vi "Create Instrument Addon From Configuration File.vi"(8 "error in (no error)":errorcluster, 10 "configuration file path":path, 11 "target in":refnum<k24>) -> (0 "error out":errorcluster, 2 "instrument addon refnum":T1=18446744073709551615 format="%.0x", 3 "target out":refnum<k24>)   [LabVIEW 2020, in "Instrument Addon Scripting API.lvlib"]
doc: "Creates an Instrument Addon and configures it according to the configuration file."
uses:
  Instrument Addon Scripting API.lvlib
  NationalInstruments.VeriStand.SystemDefinitionAPI
  <vilib>/NI VeriStand/Custom Device API/Custom Device Item Ref.ctl
  <vilib>/NI/NI VeriStand Custom Device Import and Export Tool/ImportExport.lvlib
  Addon/Addon Shared/Instrument Addon Shared.lvlib
  <vilib>/NI VeriStand/Custom Device API/Custom Device API.lvlib
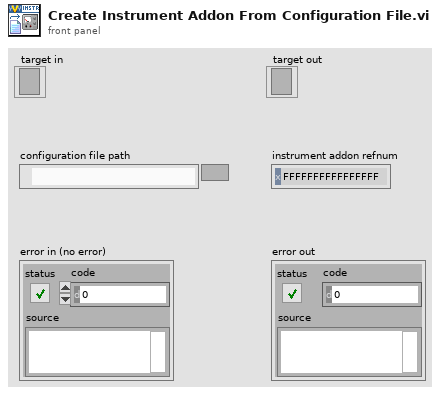
[diagram p1: front panel]
types:
  T1 = typedef "Custom Device API.lvlib/Custom Device Item Ref.ctl" = u64
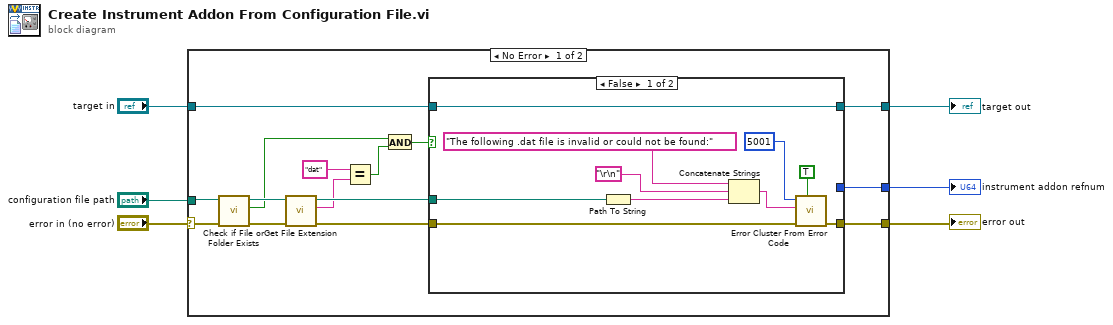
[diagram p0: block diagram]
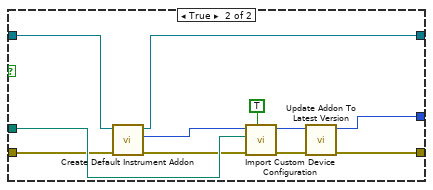
[diagram p2: hidden frame]
diagram:
  n1 = case shown="No Error" "error in (no error)" {
    selector: "error in (no error)" -> [w15 w44]
    tunnel: "target in" -> [w21 w43]
    tunnel: [w20 w43] -> w5
    tunnel: "configuration file path" -> [w13 _]
    tunnel: [w19 w44] -> w3
    tunnel: [w18 _] -> w1
    frame No Error {
      n2 = call <vilib>:"Check if File or Folder Exists.vi"("error in (no error)"=w15, "path"=w13) -> ("error out"=w14:errorcluster, "file or folder exists?"=w11:bool, "dup path"=w12:path)  [unwired: 7 in]
      n3 = call <vilib>:"Get File Extension.vi"("error in (no error)"=w14, "file"=w12) -> ("error out"=w17:errorcluster, "lowercase file extension"=w9:string, "dup file"=w16:path)  [unwired: 5 in, 2 out]
      n4 = Equal?(x="dat", y=w9) -> (x = y?=w7:bool)
      n5 = And(x=w11, y=w7) -> (x .and. y?=w10:bool)
      n6 = case shown="False" w10 {
        tunnel: w21 -> [w29 w39]
        tunnel: [w29 w38] -> w20
        tunnel: [w30 w42] -> w19
        tunnel: w17 -> [w31 w35]
        tunnel: [_ w41] -> w18
        tunnel: w16 -> [w27 w40]
        frame False {
          n7 = Path To String(path=w27) -> (string=w26:string)
          n8 = Concatenate Strings("The following .dat file is invalid or could not be found:" ("error message (\"\")"), "\r\n", w26) -> (w23:string)
          n9 = call <vilib>:"Error Cluster From Error Code.vi"("show call chain? (False)"=TRUE, "error in (no error)"=w31, "error message (\"\")"=w23, "error code (0)"=5001) -> ("error out"=w30:errorcluster)  [unwired: 5 in]
        }
        frame True {
          n10 = call "Create Default Instrument Addon.vi"("Error In"=w35, "Target In"=w39) -> ("Error Out"=w37:errorcluster, "Instrument Addon Refnum"=w36:T1, "Target Out"=w38:refnum<k24>)  [unwired: 7 in]
          n11 = call <vilib>:"Import Custom Device Configuration.vi"("Overwrite Existing?"=TRUE, "error in (no error)"=w37, "Path"=w40, "NodeID"=w36) -> ("error out"=w33:errorcluster, "NodeID out"=w34:u64)  [unwired: 5 in, 1 out]
          n12 = call "Update Addon To Latest Version.vi"("error in (no error)"=w33, "Device Item Ref in"=w34) -> ("error out"=w42:errorcluster, "Device Item Ref out"=w41:T1)  [unwired: 8 in]
        }
      }
    }
    frame Error {
    }
  }
  "target out" <- w5
  "error out" <- w3
  "instrument addon refnum" <- w1
